vi "Query Spectrum Emission Offset Sweep Mask.vi"(0 "VISA resource name":refnum<visa-resource-name>, 11 "error in (no error)":errorcluster) -> (4 "VISA resource name out":refnum<visa-resource-name>, 6 "Sweep Mode":string[](array[string]), 15 "error out":errorcluster)   [LabVIEW 2020, in "Anritsu Signal Analyzer Series.lvlib"]
doc: "Queries the sweep mode (sweep or FFT) that is executed during offset measurement in the Spectrum Emission Mask measurement."
uses:
  Anritsu Signal Analyzer Series.lvlib
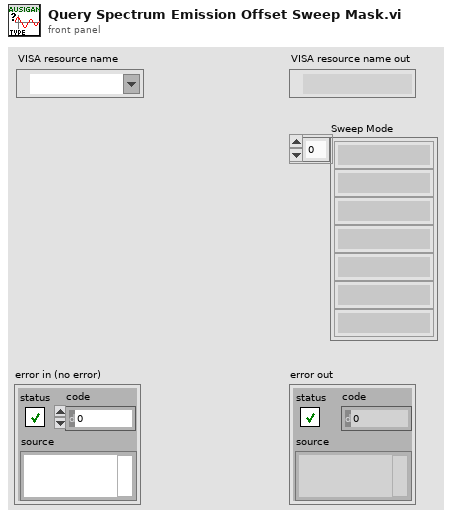
[diagram p1: front panel]
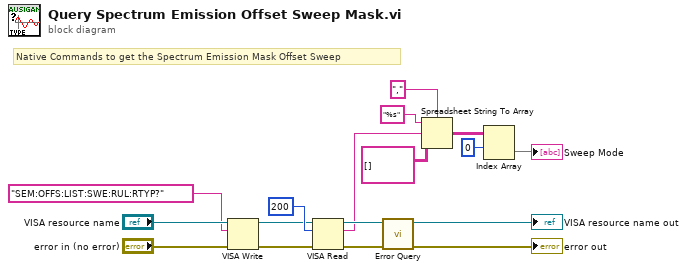
[diagram p0: block diagram]
diagram:
  # "Native Commands to get the Spectrum Emission Mask Offset Sweep"
  n1 = VISA Write(VISA resource name="VISA resource name", write buffer="SEM:OFFS:LIST:SWE:RUL:RTYP?" ("_Command"), error in (no error)="error in (no error)") -> (VISA resource name out=w11:refnum<visa-resource-name>, error out=w12:errorcluster)  [unwired: 1 out]
  n2 = VISA Read(VISA resource name=w11, byte count=u32 200 ("byte count (0)"), error in (no error)=w12) -> (VISA resource name out=w9:refnum<visa-resource-name>, read buffer=w7:string, error out=w10:errorcluster)  [unwired: 1 out]
  n3 = call "Error Query.vi"("error in (no error)"=w10, "VISA resource name"=w9) -> ("error out"=→"error out":errorcluster, "VISA resource name out"=→"VISA resource name out":refnum<visa-resource-name>)  [unwired: 6 in, 2 out]
  n4 = Spreadsheet String To Array(delimiter (Tab)=",", format string="%s", spreadsheet string=w7, array type (2D Dbl)=string[][] []) -> (array=w3:string[][])
  n5 = Index Array(array=w3, index (row)=0) -> (element=→"Sweep Mode":string[])  [unwired: 1 in]
